vi "Zero_Instruments.vi"(3 "Mode":T5, 5 "Traverse line In":T2 {"Carrier_2 Q (l/min)" format="%#.2f"; "Row Duration (mins)" format="%#.1f"; "Row No" min=0; "Trace Gas Concentration (%)" min=0.0 format="%#_4f"; "Carrier_1 Q (l/min)" format="%#.4f"; "Start X" format="%#.2f"; "Start Y" format="%#.2f"; "Start Z" format="%#.2f"; "End X" format="%#.2f"; "End Y" format="%#.2f"; "End Z" format="%#.2f"; "Tunnel Speed" format="%#.2f"; "Averaging time (mins)" min=0.0 format="%#.2f"}) -> (0 "Error Message":string, 1 "Status":T1, 2 "Traverse line Out":T2 {"Carrier_2 Q (l/min)" format="%#.2f"; "Row Duration (mins)" format="%#.1f"; "Row No" min=0; "Trace Gas Concentration (%)" min=0.0 format="%#_4f"; "Carrier_1 Q (l/min)" format="%#.4f"; "Start X" format="%#.2f"; "Start Y" format="%#.2f"; "Start Z" format="%#.2f"; "End X" format="%#.2f"; "End Y" format="%#.2f"; "End Z" format="%#.2f"; "Tunnel Speed" format="%#.2f"; "Averaging time (mins)" min=0.0 format="%#.2f"})   [LabVIEW 2022 SP3]
uses:
  Gen Trav/Traverse_cluster.ctl
  Gen Trav/Spacing.ctl
  Controls/Multi_run_mode.ctl
  Controls/User_Specific_mode.ctl
  Gen Trav/Multi_Run_Status.ctl
  Controls/Inst_type.ctl
  Controls/Setup.ctl
  Controls/Save_Data.ctl
  Camera Server/Camera enum/Camera resolution.ctl
  Globals/Meas_global.vi
panel:
  out "Zero Files":bool[](array[boolean])
  in  "permittedFailFraction":dbl=0.2 format="%#_13g"
  out "Seconds spent Total":dbl
  out "AuditTrail":string[](array[string])
  out "Seconds spent Zeroing":dbl
  out "Results":string[][](table)
  # "The Ratio should be less than 1 if the \nZero measurement is to be accepted."
  # "X           Y          Z"
  # "Start"
  # "End"
  # "X           Y          Z"
  # "Start"
  # "End"
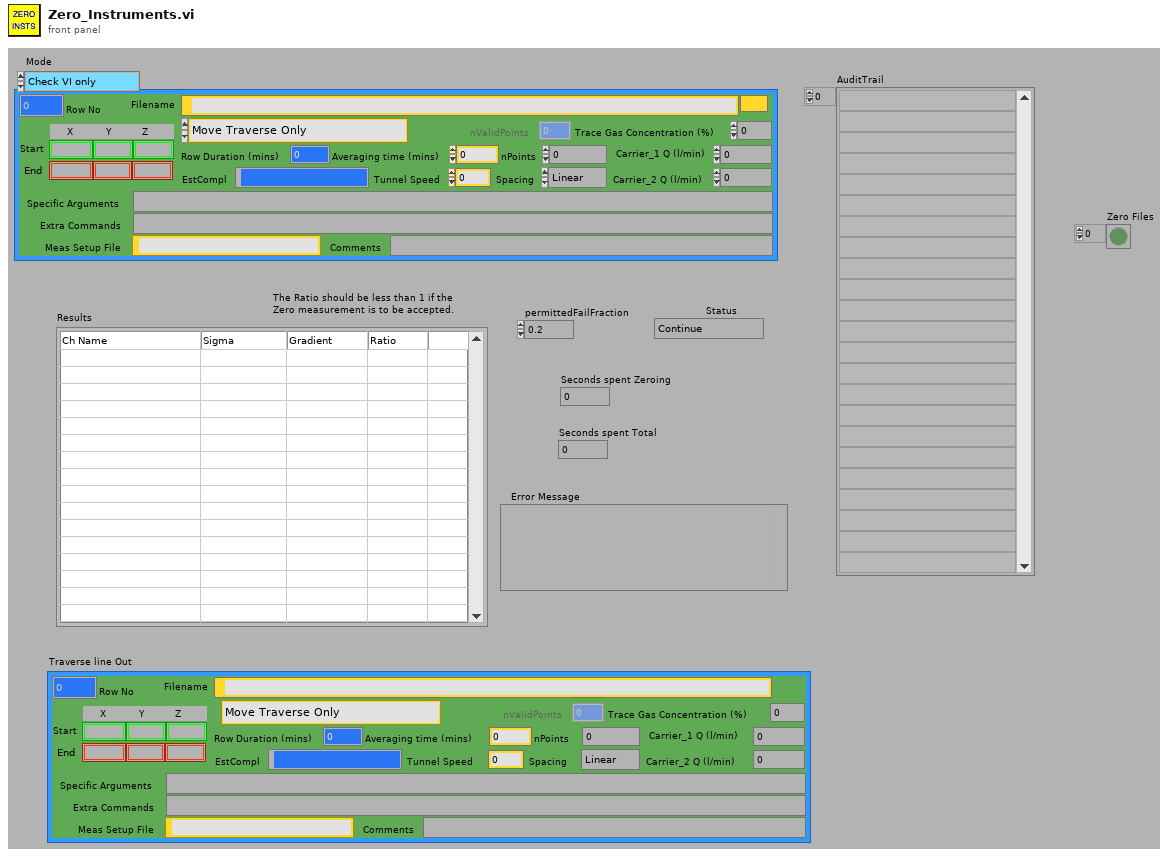
[diagram p1: front panel]
types:
  T1 = typedef "Multi_Run_Status.ctl" = enum16{"Continue", "Continue with Error", "Jump to Next Point", "Jump to Next Row", "Jump To Fall Back", "Terminate Run"}
  T2 = typedef "Traverse_cluster.ctl" = cluster{"Start X":sgl, "Start Y":sgl, "Start Z":sgl, "End X":sgl, "End Y":sgl, "End Z":sgl, "nPoints":i32, "Spacing":T3, "Filename":path, "Tunnel Speed":dbl, "Averaging time (mins)":dbl, "Extra Commands":string, "Carrier_1 Q (l/min)":dbl, "Carrier_2 Q (l/min)":dbl, "Trace Gas Concentration (%)":dbl, "Specific Arguments":string, "Comments":string, "Row No":i32, "Row Type Selector":T4, "EstCompl":string, "Row Duration (mins)":dbl, "nValidPoints":i32, "Meas Setup File":string}
  T3 = typedef "Spacing.ctl" = enum16{"Linear", "Log", "Gauss", "Specified", "N/A"}
  T4 = typedef "Multi_run_mode.ctl" = enum16{"Move Traverse Only", "Set Tunnel Speed Only", "Set Source Only", "Set Measurement Conditions", "Single Measurement", "Vertical Profile", "Lateral Profile", "Longitudinal Profile", "Multi-Axis Profile", "Explore Volume", "Auto Calibrate", "Meas Fast FID Bkgnd", "Check Beam Power", "Scanning Valve Measurement", "Run VI Named:", "Set ADAM Ch", "Wait (minutes)", "Send Message", "Synchronize With:", "Fall Back to this Row", "Turn Off Row Repeating", "Traverse 3D Volume", "Blank Row", "Jump to Fall Back Row"}
  T5 = typedef "User_Specific_mode.ctl" = enum16{"Check VI only", "Run VI"}
  T6 = typedef "Inst_type.ctl" = enum16{"Raw voltage", "Raw with zero offsetting", "Propeller anemometer", "Pressure Transducer", "Pitot-static tube", "Hot wire", "Cross wire 1", "Cross wire 2", "Generic Linear", "Generic Polynomial", "Generic BackPoly", "Fast FID", "Thermocouple", "Cold wire", "Pulsed Wire", "LDA Vel", "LDA Tran time", "LDA Arr time", "Microphone"}
  T7 = typedef "Save_Data.ctl" = enum16{"Save No Data", "Save Data"}
  T8 = typedef "Setup.ctl" = enum16{"Run Program", "Show Setup", "Save Current Setup", "Setup Front Panel"}
  T9 = typedef "Analysis_info_cluster.ctl" = cluster{"Colour":u32, "Inst type":T6, "Inst name":string, "Symbol":string, "Code name":string, "Extra Info":string, "Inst Array":T10, "U":dbl, "u^2":dbl, "u^3":dbl, "u^4":dbl, "Skew_u":dbl, "Kurt_u":dbl, "Sd Error in Mean":dbl, "% u'/U":dbl, "X":dbl, "Y":dbl, "Z":dbl, "Timescale integral Estimate":dbl, "Sd Error in Variance":dbl, "Calib File":path, "Calib Constants":dbl[], "Output Position":bool, "Stats":enum16{"None", "Basic", "Full"}, "Av Sampling Rate":dbl, "Av No of Samples":dbl, "Total Meas Time (s)":dbl, "OrigChName":string, "Max value":dbl, "Min value":dbl, "Req Sample Rate Hz":dbl, "Sync Delay Time (s)":dbl, "Ch No":i16, "Device":string, "Use Latest Calib":bool, "Port":string, "Metadata Ch Names":string[], "Metadata Ch Values":string[], "Label":string, "chState":T11, "Point Drift":dbl, "inputConfig":string}
  T10 = typedef "Instrument_Array.ctl" = enum16{"PWA", "LDA", "Analogue"}
  T11 = typedef "channelState.ctl" = enum32{"No Selection", "Solo", "Mute"}
  T12 = typedef "Time_Trace_Cluster.ctl" = cluster{"Weighting":dbl[], "Voltage":dbl[], "Eng Values":dbl[]}
  T13 = typedef "Camera resolution.ctl" = u8
  T14 = typedef "Data for Inst Type.ctl" = enum16{"Eng Values", "Voltage"}
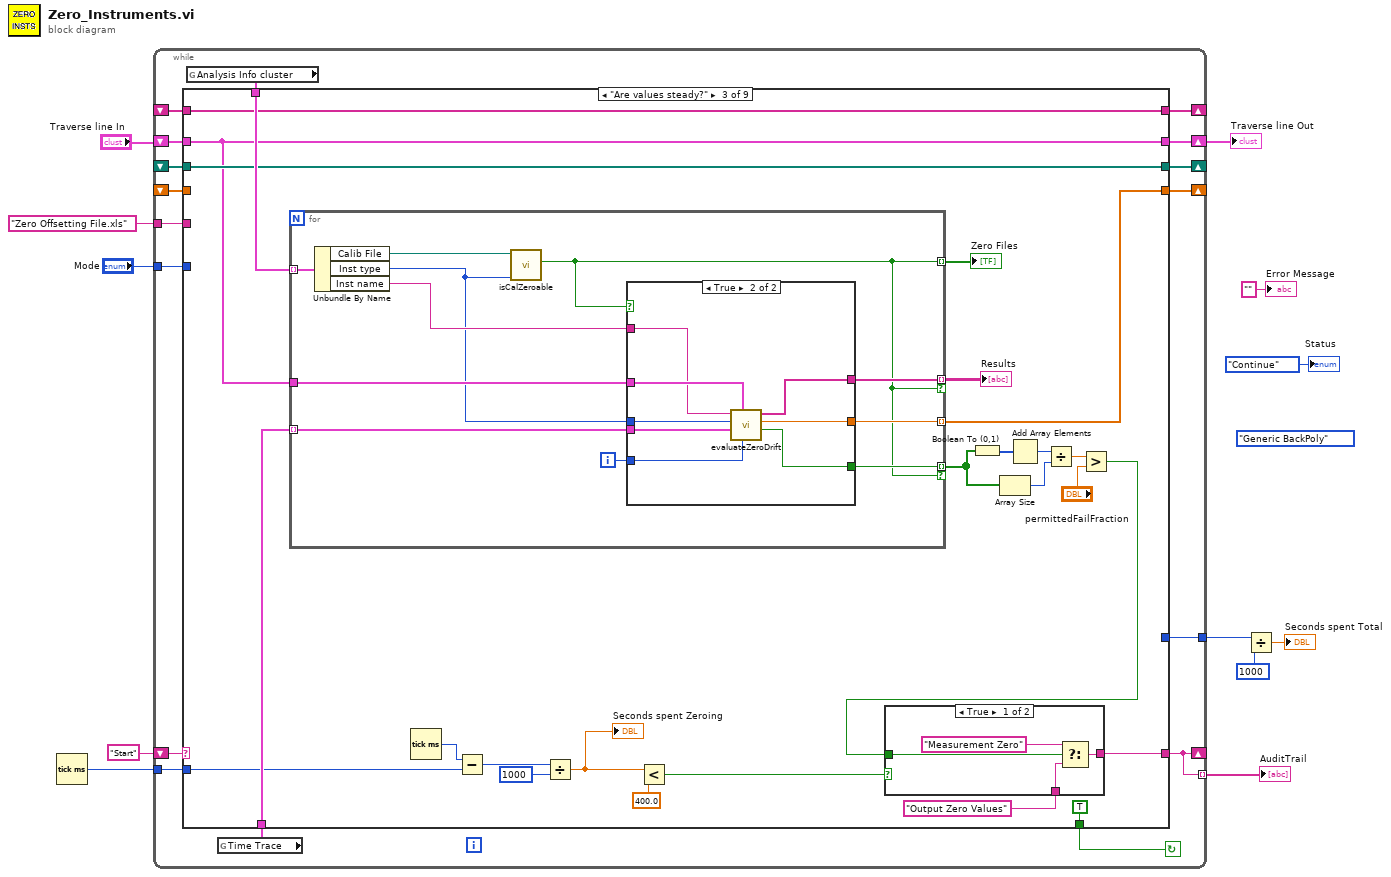
[diagram p0: block diagram]
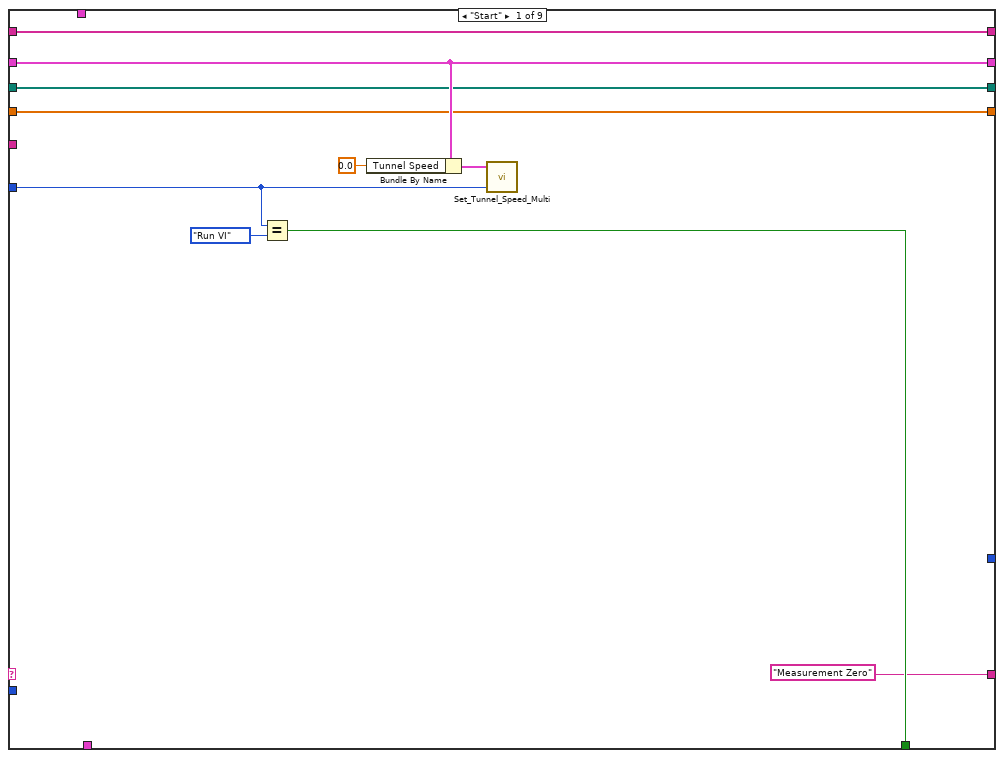
[diagram p2: hidden frame]
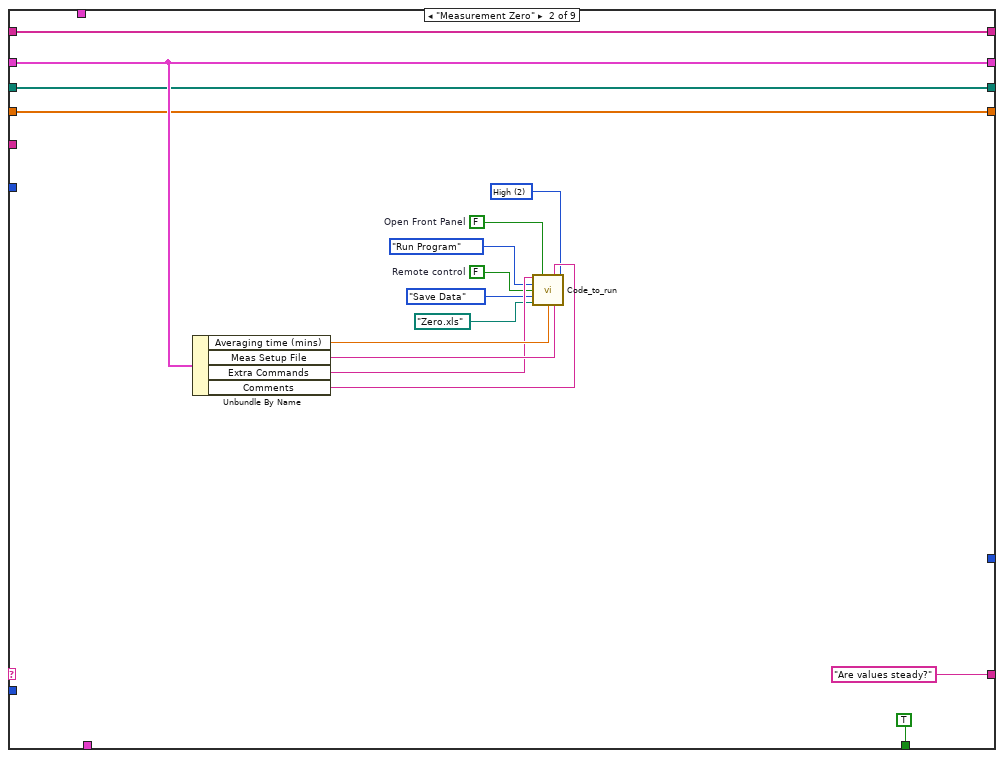
[diagram p3: hidden frame]
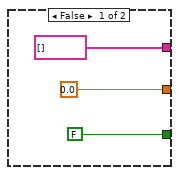
[diagram p4: hidden frame]
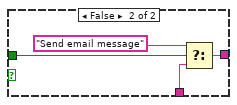
[diagram p5: hidden frame]
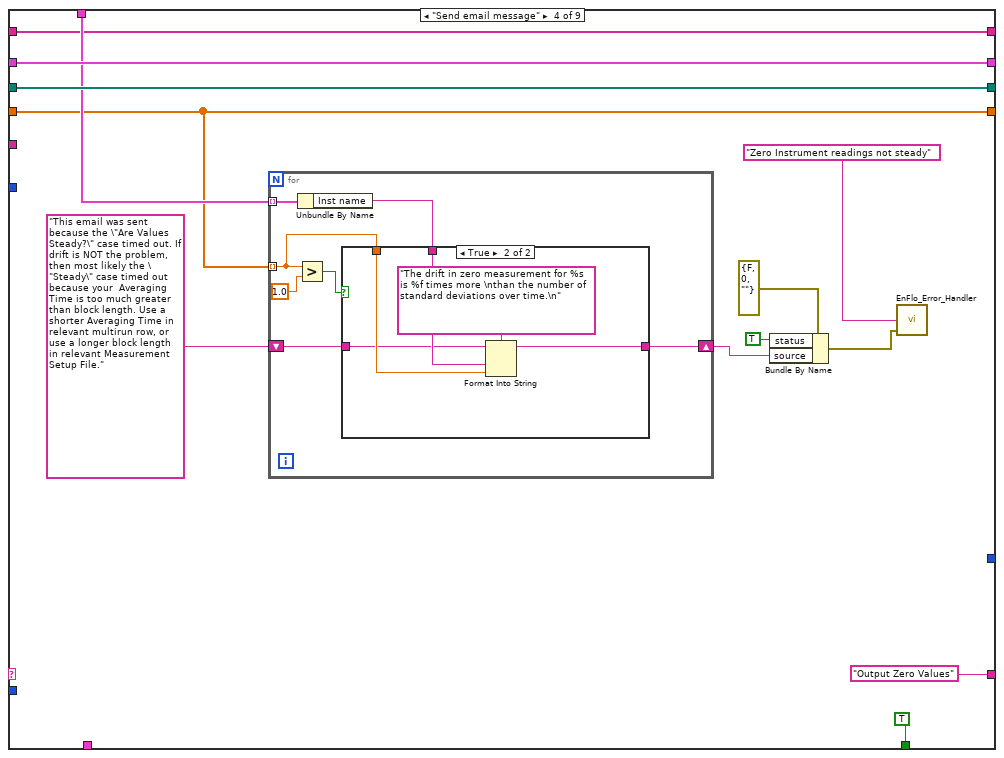
[diagram p6: hidden frame]
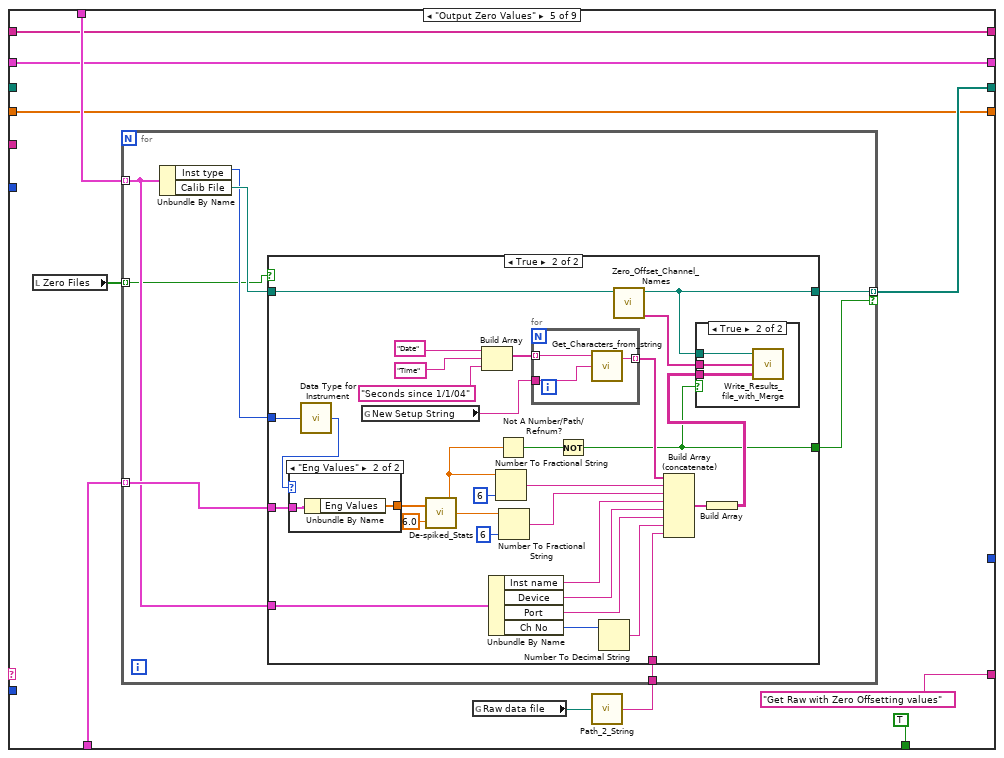
[diagram p8: hidden frame]
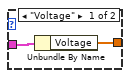
[diagram p10: hidden frame]
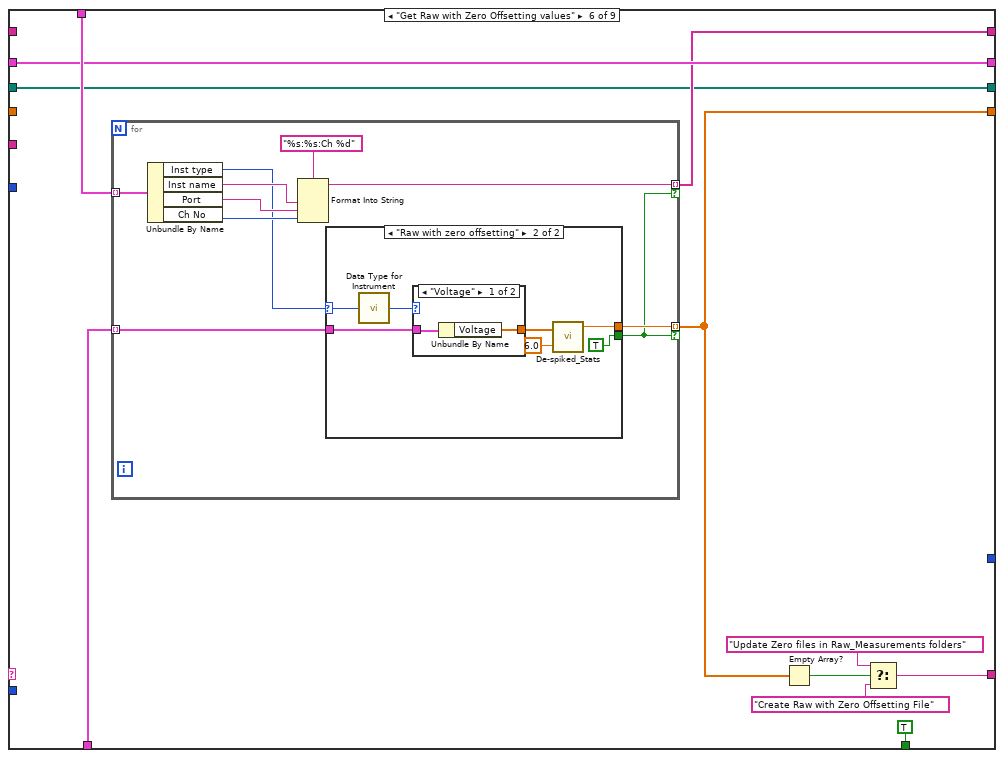
[diagram p12: hidden frame]
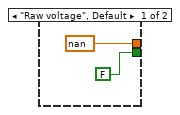
[diagram p13: hidden frame]
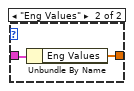
[diagram p14: hidden frame]
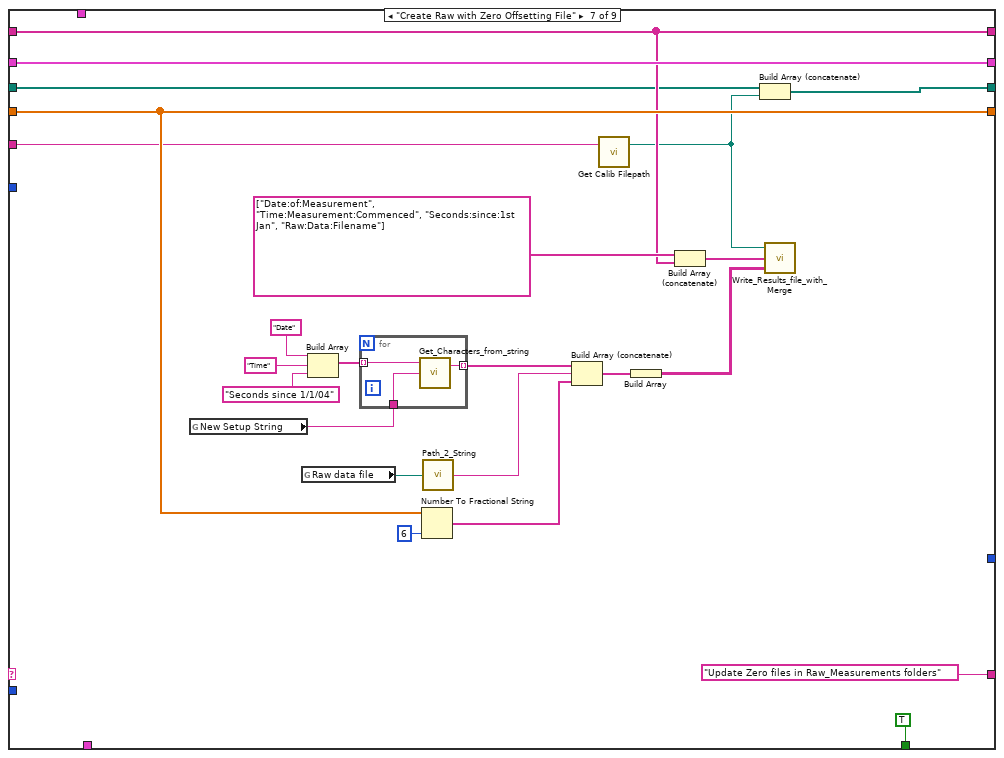
[diagram p15: hidden frame]
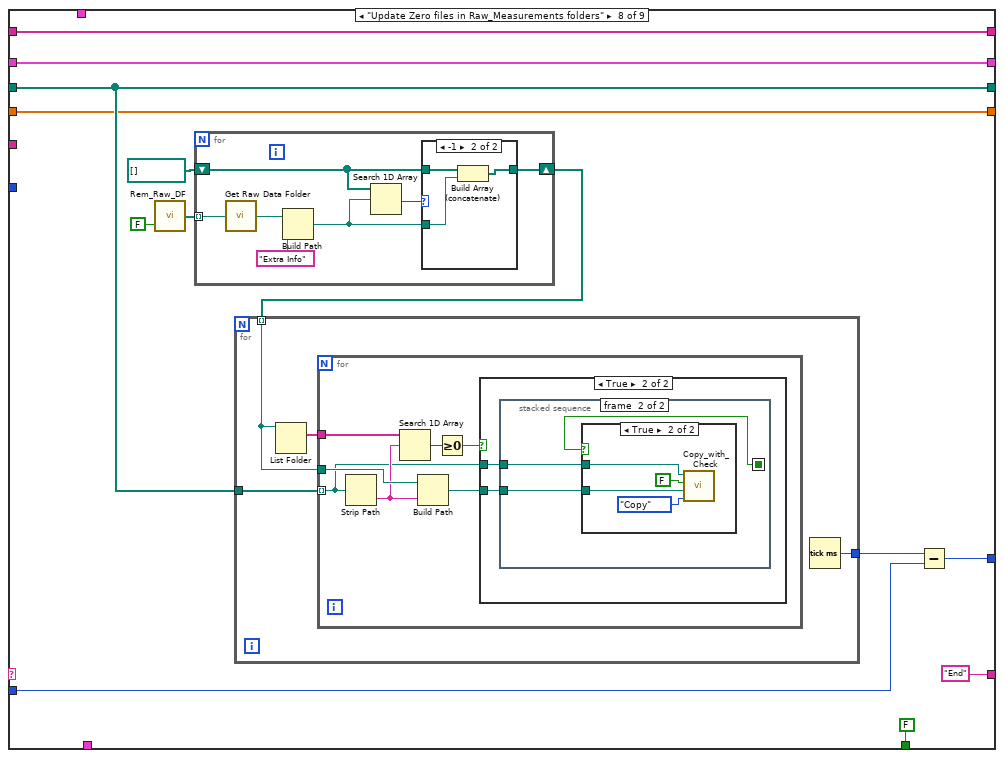
[diagram p16: hidden frame]
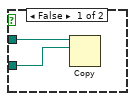
[diagram p17: hidden frame]
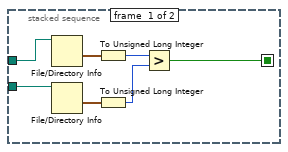
[diagram p18: hidden frame]
diagram:
  (unwired) Inst_type."Generic BackPoly" ("Inst type")
  n1 = Tick Count (ms)() -> (millisecond timer value=w7:u32)
  n2 = while {
    shift-right: [w18] -> _
    shift-left: "Start" -> [w14]
    shift-right: [w26] -> w11
    shift-left: "Traverse line In" -> [w28]
    tunnel: "Mode" -> [w27]
    tunnel: w7 -> [w23]
    shift-right: [w22] -> _
    shift-left: _ -> [w21]
    shift-right: [w20] -> _
    shift-left: _ -> [w19]
    tunnel: [w18] -> w6 mode=indexing
    shift-right: [w17] -> _
    shift-left: _ -> [w16]
    tunnel: "Zero Offsetting File.xls" ("Filename String") -> [w15]
    tunnel: [w13] -> w3
    stop <- w29 continue-if-true
    n3 = global read "Meas_global.vi" "Analysis Info cluster"() -> (w24:T9[])
    n4 = global read "Meas_global.vi" "Time Trace"() -> (w25:T12[])
    n5 = case shown="\"Are values steady?\"" w14 {
      selector: w14 -> [_ _ _ _ _ _ _ _ w312]
      tunnel: [w34 TRUE TRUE TRUE TRUE TRUE TRUE FALSE FALSE] -> w29
      tunnel: w28 -> [w37 w54 w58 w122 w144 w207 w245 w271 w316]
      tunnel: w27 -> [w36 _ _ _ _ _ _ _ _]
      tunnel: [w37 w54 w58 w122 w144 w207 w245 w271 w316] -> w26
      tunnel: ["Measurement Zero" "Are values steady?" w76 "Output Zero Values" "Get Raw with Zero Offsetting values" w202 "Update Zero files in Raw_Measurements folders" "End" "End"] -> w18
      tunnel: w25 -> [_ _ w79 _ w146 w209 _ _ _]
      tunnel: w24 -> [_ _ w78 w120 w145 w208 _ _ _]
      tunnel: w23 -> [_ _ w74 _ _ _ _ w260 _]
      tunnel: [w32 w52 w73 w121 w140 w204 w235 w266 w315] -> w22
      tunnel: w21 -> [w32 w52 w73 w121 _ w204 w237 w266 w315]
      tunnel: [w31 w51 w70 w118 w138 w206 w244 w263 w314] -> w20
      tunnel: w19 -> [w31 w51 _ w118 w138 _ w244 w263 w314]
      tunnel: [w30 w50 w59 w116 w139 w205 w243 w262 w313] -> w17
      tunnel: w16 -> [w30 w50 w59 w116 w139 _ w243 w262 w313]
      tunnel: w15 -> [_ _ _ _ _ _ w234 _ _]
      tunnel: [_ _ _ _ _ _ _ w259 _] -> w13
      frame "Start" {
        n6 = Equal?(x=w36, y=User_Specific_mode."Run VI") -> (x = y?=w34:bool)
        n7 = Bundle By Name(cluster=w37, "Tunnel Speed"=0.0) -> (w39:T2)
        n8 = call "Set_Tunnel_Speed_Multi.vi"("Simulate/Run"=w36, "Traverse line"=w39) -> ()  [unwired: 4 out]
      }
      frame "Measurement Zero" {
        w44 = T13 2 items=["Low", "Med.", "High", "Max."] ("Camera Resolution")
        w45 = FALSE  # Open Front Panel
        w42 = FALSE  # Remote control
        n9 = Unbundle By Name(w54) -> ("Averaging time (mins)"=w49:dbl, "Meas Setup File"=w48:string, "Extra Commands"=w47:string, "Comments"=w46:string)
        n10 = call "Code_to_run.vi"("Extra command String"=w47, "Open Front Panel"=w45, "Current Row Comments"=w46, "Camera Resolution"=w44, "setup"=Setup."Run Program", "Remote control"=w42, "File"=Save_Data."Save Data", "Results Filename"=path "Zero.xls" ("Filename"), "Averaging time (min)"=w49, "Setup filename"=w48) -> ()  [unwired: 2 in, 4 out]
      }
      frame "Are values steady?" {
        n11 = for {
          tunnel: w78 -> [w91] mode=indexing
          tunnel: w79 -> [w90] mode=indexing
          tunnel: [w89] -> w65 mode=indexing if=w82
          tunnel: [w88] -> w70 mode=indexing
          tunnel: [w87] -> w69 mode=indexing if=w82
          tunnel: w58 -> [w85]
          tunnel: [w82] -> w56 mode=indexing
          i -> [w86]
          n12 = Unbundle By Name(w91) -> ("Calib File"=w84:path, "Inst type"=w81:T6, "Inst name"=w83:string)
          n13 = call "isCalZeroable.vi"("Inst type"=w81, "Calib File"=w84) -> ("Zeroable?"=w82:bool)  [unwired: 9 in]
          n14 = case shown="True" w82 {
            tunnel: w90 -> [_ w102]
            tunnel: [FALSE w99] -> w89
            tunnel: [0.0 w100] -> w88
            tunnel: [string[] [] w101] -> w87
            tunnel: w81 -> [_ w98]
            tunnel: w86 -> [_ w97]
            tunnel: w85 -> [_ w96]
            tunnel: w83 -> [_ w95]
            frame False {
            }
            frame True {
              n15 = call "evaluateZeroDrift.vi"("chIndex"=w97, "Traverse line In"=w96, "Time Trace"=w102, "Inst type"=w98, "Inst name"=w95) -> ("Drifty?"=w99:bool, "ratio"=w100:dbl, "tableRow"=w101:string[])  [unwired: 4 in]
            }
          }
        }
        "Results" <- w69
        "Zero Files" <- w56
        n16 = Tick Count (ms)() -> (millisecond timer value=w75:u32)
        n17 = Subtract(x=w75, y=w74) -> (x-y=w68:u32)
        n18 = Divide(x=w68, y=u32 1000) -> (x/y=w57:dbl)
        "Seconds spent Zeroing" <- w57
        n19 = Less?(x=w57, y=400.0) -> (x < y?=w72:bool)
        n20 = Boolean To (0,1)(Boolean=w65) -> (0, 1=w66:i16[])
        n21 = Array Size(array=w65) -> (size(s)=w63:i32)
        n22 = Add Array Elements(numeric array=w66) -> (sum=w64:i16)
        n23 = Divide(x=w64, y=w63) -> (x/y=w62:dbl)
        n24 = Greater?(x=w62, y="permittedFailFraction") -> (0:w60:bool)
        n25 = case shown="True" w72 {
          tunnel: [w106 w110] -> w76
          tunnel: w60 -> [w104 w109]
          tunnel: "Output Zero Values" -> [w103 w107]
          frame True {
            n26 = Select(t="Measurement Zero", s=w104, f=w103) -> (s? t:f=w106:string)
          }
          frame False {
            n27 = Select(t="Send email message", s=w109, f=w107) -> (s? t:f=w110:string)
          }
        }
      }
      frame "Send email message" {
        n28 = for {
          tunnel: w120 -> [w130] mode=indexing
          tunnel: w118 -> [w126] mode=indexing
          shift-right: [w124] -> w113
          shift-left: "This email was sent because the \"Are Values Steady?\" case timed out. If drift is NOT the problem, then most likely the \"Steady\" case timed out because your  Averaging Time is too much greater than block length. Use a shorter Averaging Time in relevant multirun row, or use a longer block length in relevant Measurement Setup File." -> [w125]
          n29 = Greater?(x=w126, y=1.0) -> (0:w128:bool)
          n30 = Unbundle By Name(w130) -> ("Inst name"=w127:string)
          n31 = case shown="True" w128 {
            tunnel: w127 -> [_ w136]
            tunnel: w126 -> [_ w135]
            tunnel: w125 -> [w131 w134]
            tunnel: [w131 w133] -> w124
            frame False {
            }
            frame True {
              n32 = Format Into String(format string="The drift in zero measurement for %s is %f times more \nthan the number of standard deviations over time.\n", initial string=w134, w136, w135) -> (resulting string=w133:string)  [unwired: 1 in, 1 out]
            }
          }
        }
        n33 = Bundle By Name(cluster=errorcluster {"status"=FALSE, "code"=0, "source"=""} ("error in (no error)"), "status"=TRUE, "source"=w113) -> (w112:errorcluster)
        n34 = call "EnFlo_Error_Handler.vi"("error in (no error)"=w112, "Error Type"="Zero Instrument readings not steady") -> ()  [unwired: 2 in, 2 out]
      }
      frame "Output Zero Values" {
        n35 = local read "Zero Files"() -> (w137:bool[])
        n36 = global read "Meas_global.vi" "Raw data file"() -> (w142:path)
        n37 = call "Path_2_String.vi"("Real Path"=w142) -> ("Path String"=w141:string)
        n38 = for {
          tunnel: w145 -> [w151] mode=indexing
          tunnel: w146 -> [w155] mode=indexing
          tunnel: w141 -> [w154]
          tunnel: [w153] -> w140 mode=indexing if=w152
          tunnel: w137 -> [w148] mode=indexing
          n39 = Unbundle By Name(w151) -> ("Inst type"=w149:T6, "Calib File"=w150:path)
          n40 = case shown="True" w148 {
            selector: w148 -> [w156 _]
            tunnel: w155 -> [_ w160]
            tunnel: w154 -> [_ w163]
            tunnel: w150 -> [w157 w173]
            tunnel: [w157 w172] -> w153
            tunnel: [w156 w169] -> w152
            tunnel: w151 -> [_ w161]
            tunnel: w149 -> [_ w158]
            frame False {
            }
            frame True {
              n41 = call "Data Type for Instrument.vi"("Inst type"=w158) -> ("Data for Inst Type"=w162:T14)
              n42 = case shown="\"Eng Values\"" w162 {
                tunnel: [w190 w192] -> w159
                tunnel: w160 -> [w189 w191]
                frame "Voltage" {
                  n43 = Unbundle By Name(w189) -> ("Voltage"=w190:dbl[])
                }
                frame "Eng Values" {
                  n44 = Unbundle By Name(w191) -> ("Eng Values"=w192:dbl[])
                }
              }
              n45 = global read "Meas_global.vi" "New Setup String"() -> (w180:string)
              n46 = call "De-spiked_Stats.vi"("Raw Signal"=w159, "No of st dev to chop at"=6.0) -> ("mean"=w171:dbl, "standard deviation"=w185:dbl)  [unwired: 1 out]
              n47 = Build Array("Date", "Time", "Seconds since 1/1/04") -> (w181:string[])
              n48 = Unbundle By Name(w161) -> ("Inst name"=w168:string, "Device"=w167:string, "Port"=w166:string, "Ch No"=w165:i16)
              n49 = Number To Fractional String(number=w171, precision (6)=i16 6) -> (F-format string=w178:string)  [unwired: 2 out]
              n50 = Not A Number/Path/Refnum?(number/path/refnum=w171) -> (NaN/Path/Refnum?=w170:bool)
              n51 = Number To Fractional String(number=w185, precision (6)=i16 6) -> (F-format string=w177:string)  [unwired: 2 out]
              n52 = for {
                tunnel: w181 -> [w198] mode=indexing
                tunnel: w180 -> [w197]
                tunnel: [w196] -> w179 mode=indexing
                n53 = call "Get_Characters_from_string.vi"("Input string"=w197, "Variable name"=w198) -> ("Value"=w196:string)  [unwired: 1 in, 1 out]
              }
              n54 = Not(x=w170) -> (.not. x?=w169:bool)
              n55 = Number To Decimal String(number=w165) -> (decimal integer string=w164:string)  [unwired: 1 in]
              n56 = call "Zero_Offset_Channel_Names.vi"("Calib Filename"=w173) -> ("Channel names"=w176:string[], "Zero Filename"=w172:path)  [unwired: 3 in, 2 out]
              n57 = Build Array (concatenate)(w179, w178, w177, w168, w167, w166, w164, w163) -> (w175:string[])
              n58 = Build Array(w175) -> (w174:string[][])
              n59 = case shown="True" w169 {
                tunnel: w176 -> [_ w194]
                tunnel: w174 -> [_ w193]
                tunnel: w172 -> [_ w195]
                frame False {
                }
                frame True {
                  n60 = call "Write_Results_file_with_Merge.vi"("Values In"=w193, "Channel Names in"=w194, "Filename"=w195) -> ()  [unwired: 1 in, 2 out]
                }
              }
            }
          }
        }
      }
      frame "Get Raw with Zero Offsetting values" {
        n61 = for {
          tunnel: w208 -> [w218] mode=indexing
          tunnel: w209 -> [w219] mode=indexing
          tunnel: [w217] -> w206 mode=indexing if=w216
          tunnel: [w214] -> w205 mode=indexing if=w216
          n62 = Unbundle By Name(w218) -> ("Inst type"=w210:T6, "Inst name"=w215:string, "Port"=w213:string, "Ch No"=w212:i16)
          n63 = Format Into String(format string="%s:%s:Ch %d", w215, w213, w212) -> (resulting string=w214:string)  [unwired: 2 in, 1 out]
          n64 = case shown="\"Raw with zero offsetting\"" w210 {
            selector: w210 -> [_ w222]
            tunnel: w219 -> [_ w224]
            tunnel: [FALSE TRUE] -> w216
            tunnel: [nan ("mean") w226] -> w217
            frame "Raw voltage", Default {
            }
            frame "Raw with zero offsetting" {
              n65 = call "Data Type for Instrument.vi"("Inst type"=w222) -> ("Data for Inst Type"=w225:T14)
              n66 = case shown="\"Voltage\"" w225 {
                tunnel: [w230 w232] -> w223
                tunnel: w224 -> [w229 w231]
                frame "Voltage" {
                  n67 = Unbundle By Name(w229) -> ("Voltage"=w230:dbl[])
                }
                frame "Eng Values" {
                  n68 = Unbundle By Name(w231) -> ("Eng Values"=w232:dbl[])
                }
              }
              n69 = call "De-spiked_Stats.vi"("Raw Signal"=w223, "No of st dev to chop at"=6.0) -> ("mean"=w226:dbl)  [unwired: 2 out]
            }
          }
        }
        n70 = Empty Array?(array=w206) -> (empty?=w200:bool)
        n71 = Select(t="Update Zero files in Raw_Measurements folders", s=w200, f="Create Raw with Zero Offsetting File") -> (s? t:f=w202:string)
      }
      frame "Create Raw with Zero Offsetting File" {
        n72 = global read "Meas_global.vi" "New Setup String"() -> (w254:string)
        n73 = global read "Meas_global.vi" "Raw data file"() -> (w240:path)
        n74 = Build Array("Date", "Time", "Seconds since 1/1/04") -> (w255:string[])
        n75 = for {
          tunnel: w255 -> [w258] mode=indexing
          tunnel: w254 -> [w257]
          tunnel: [w256] -> w249 mode=indexing
          n76 = call "Get_Characters_from_string.vi"("Input string"=w257, "Variable name"=w258) -> ("Value"=w256:string)  [unwired: 1 in, 1 out]
        }
        n77 = Number To Fractional String(number=w244, precision (6)=i16 6) -> (F-format string=w238:string[])  [unwired: 2 out]
        n78 = call "Path_2_String.vi"("Real Path"=w240) -> ("Path String"=w239:string)
        n79 = Build Array (concatenate)(w249, w239, w238) -> (w247:string[])
        n80 = call "Get Calib Filepath.vi"("Filename String"=w234) -> ("Filename Out"=w236:path)  [unwired: 2 in]
        n81 = Build Array(w247) -> (w246:string[][])
        n82 = Build Array (concatenate)(string[] ["Date:of:Measurement", "Time:Measurement:Commenced", "Seconds:since:1st Jan", "Raw:Data:Filename"] ("Channel names"), w243) -> (w248:string[])
        n83 = Build Array (concatenate)(w237, w236) -> (w235:path[])
        n84 = call "Write_Results_file_with_Merge.vi"("Values In"=w246, "Channel Names in"=w248, "Filename"=w236) -> ()  [unwired: 1 in, 2 out]
      }
      frame "Update Zero files in Raw_Measurements folders" {
        n85 = call "Rem_Raw_DF.vi"("Clear History?"=FALSE) -> ("List of Filenames"=w269:path[])  [unwired: 1 in]
        n86 = for {
          tunnel: w269 -> [w302] mode=indexing
          shift-right: [w305] -> w267
          shift-left: path[] [] -> [w306]
          n87 = call "Get Raw Data Folder.vi"("Raw data file"=w302) -> ("Main Raw Data Folder"=w304:path)
          n88 = Build Path(base path=w304, name or relative path="Extra Info") -> (appended path=w301:path)
          n89 = Search 1D Array(1D array=w306, element=w301) -> (index of element=w307:i32)  [unwired: 1 in]
          n90 = case shown="-1" w307 {
            tunnel: w306 -> [w308 w311]
            tunnel: w301 -> [_ w310]
            tunnel: [w308 w309] -> w305
            frame Default {
            }
            frame -1 {
              n91 = Build Array (concatenate)(w311, w310) -> (w309:path[])
            }
          }
        }
        n92 = for {
          tunnel: w267 -> [w274] mode=indexing
          tunnel: w266 -> [w273]
          tunnel: [w272] -> w261
          n93 = List Folder(path=w274) -> (filenames=w275:string[])  [unwired: 1 in, 5 out]
          n94 = for {
            tunnel: w273 -> [w276] mode=indexing
            tunnel: w274 -> [w279]
            tunnel: w275 -> [w282]
            n95 = Strip Path(path=w276) -> (name=w278:string)  [unwired: 1 out]
            n96 = Search 1D Array(1D array=w282, element=w278) -> (index of element=w281:i32)  [unwired: 1 out]
            n97 = Build Path(base path=w279, name or relative path=w278) -> (appended path=w277:path)
            n98 = Greater Or Equal To 0?(x=w281) -> (x >= 0?=w280:bool)
            n99 = case shown="True" w280 {
              tunnel: w277 -> [w284 w285]
              tunnel: w276 -> [w283 w286]
              frame False {
                n100 = Copy(10:w284, 11:w283) -> ()  [unwired: 1 in, 5 out]
              }
              frame True {
                n101 = stacked-sequence {
                  seq-local: [w289 _] -> [_ w296]
                  tunnel: w286 -> [w293 w294]
                  tunnel: w285 -> [w292 w295]
                  frame #0 {
                    n102 = File/Directory Info(path=w293) -> (last mod=w287:timestamp)  [unwired: 1 in, 6 out]
                    n103 = File/Directory Info(path=w292) -> (last mod=w288:timestamp)  [unwired: 1 in, 6 out]
                    n104 = To Unsigned Long Integer(number=w287) -> (unsigned 32bit integer=w291:u32)
                    n105 = To Unsigned Long Integer(number=w288) -> (unsigned 32bit integer=w290:u32)
                    n106 = Greater?(x=w291, y=w290) -> (0:w289:bool)
                  }
                  frame #1 {
                    n107 = case shown="True" w296 {
                      tunnel: w295 -> [_ w299]
                      tunnel: w294 -> [_ w300]
                      frame False {
                      }
                      frame True {
                        n108 = call "Copy_with_Check.vi"("Mode"=enum16{"Move", "Copy"}."Copy", "Target Path"=w299, "Variable Target?"=FALSE, "Source Path"=w300) -> ()  [unwired: 1 out]
                      }
                    }
                  }
                }
              }
            }
          }
          n109 = Tick Count (ms)() -> (millisecond timer value=w272:u32)
        }
        n110 = Subtract(x=w261, y=w260) -> (x-y=w259:u32)
      }
      frame Default {
        n111 = call "Case not matched.vi"("Case Name not Matched"=w312) -> ()
      }
    }
  }
  "Traverse line Out" <- w11
  "AuditTrail" <- w6
  n112 = Divide(x=w3, y=u32 1000) -> (x/y=→"Seconds spent Total":dbl)
  "Error Message" <- "" ("Error Message")
  "Status" <- Multi_Run_Status."Continue" ("Status")
